vi "ConfigureIndex.vi"(0 "Axis In":T7, 1 "Additional Settings":T4={"Next Index"=0, "Termination"=0, "Count"=1} {"Termination" items=["Stop", "Start Another Immediately", "Start Another x/start Index Input", "Start Another Index Without Stopping"]}, 5 "Index (0)":T6, 7 "Position":dbl, 11 "error in (no error)":errorcluster, 12 "Index Settings":T1={"Type"=1, "Dwell"=0, "Velocity"=0.0, "Accel/Decel"=0.0} {"Type" items=["Incremental", "Absolute", "Registration", "Jog"]}) -> (4 "Axis Out":T7, 6 "Index (duplicate)":T6, 15 "error out":errorcluster)   [LabVIEW 2009]
doc: "Configure an index (motion) on specified axis. Any parameters left unset will be set to their default values."
uses:
  typedefs/AxisSelect_Enum.ctl
  typedefs/Ultra3000/Index_Numeric.ctl
  typedefs/Ultra3000/AdditionalIndexSettings_Cluster.ctl
  typedefs/Ultra3000/IndexTermination.ctl
  typedefs/Ultra3000/IndexSettings_Cluster.ctl
  typedefs/Ultra3000/IndexType.ctl
  typedefs/DwellTime.ctl
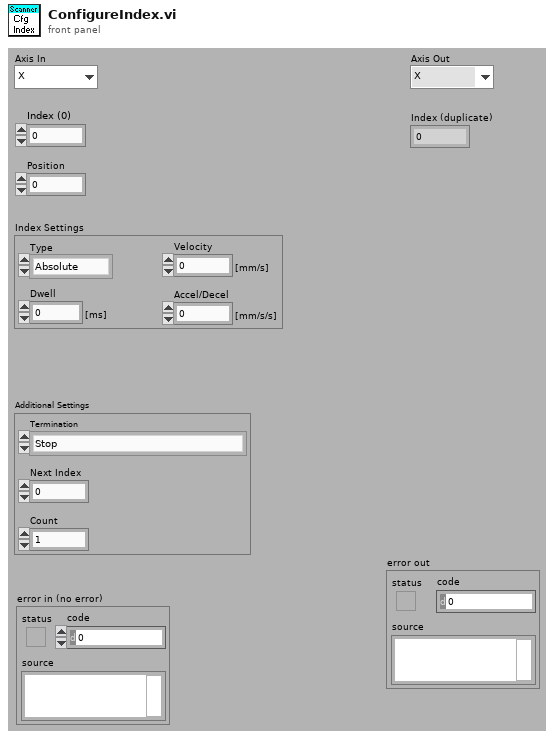
[diagram p1: front panel]
types:
  T1 = typedef "IndexSettings_Cluster.ctl" = cluster{"Type":T2, "Dwell":T3, "Velocity":dbl, "Accel/Decel":dbl}
  T2 = typedef "IndexType.ctl" = i32
  T3 = typedef "DwellTime.ctl" = u16
  T4 = typedef "AdditionalIndexSettings_Cluster.ctl" = cluster{"Next Index":u8, "Termination":T5, "Count":u16}
  T5 = typedef "IndexTermination.ctl" = i32
  T6 = typedef "Index_Numeric.ctl" = u8
  T7 = typedef "AxisSelect_Enum.ctl" = enum16{"X", "Y", "Z", "Axis Space"}
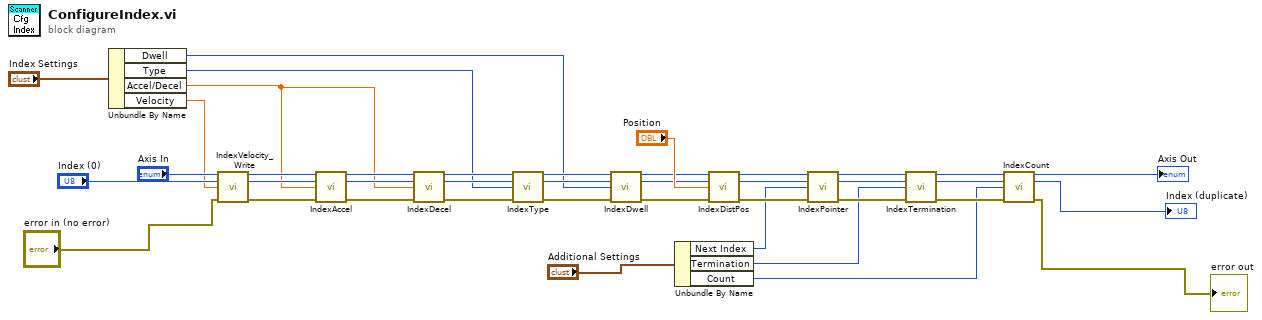
[diagram p0: block diagram]
diagram:
  n1 = Unbundle By Name("Index Settings") -> ("Dwell"=w6:T3, "Type"=w19:T2, "Accel/Decel"=w20:dbl, "Velocity"=w21:dbl)
  n2 = call "IndexVelocity_Write.vi"("Axis In"="Axis In", "Index (0)"="Index (0)", "Velocity"=w21, "error in (no error)"="error in (no error)") -> ("Axis Out"=w29:T7, "Index (duplicate)"=w26:T6, "error out"=w36:errorcluster)  [unwired: 9 in]
  n3 = call "IndexAccel.vi"("Axis In"=w29, "Index (0)"=w26, "Acceleration"=w20, "error in (no error)"=w36) -> ("Axis Out"=w30:T7, "Index (duplicate)"=w25:T6, "error out"=w37:errorcluster)  [unwired: 9 in]
  n4 = call "IndexDecel.vi"("Axis In"=w30, "Index (0)"=w25, "Deceleration"=w20, "error in (no error)"=w37) -> ("Axis Out"=w31:T7, "Index (duplicate)"=w24:T6, "error out"=w38:errorcluster)  [unwired: 9 in]
  n5 = call "IndexType.vi"("Axis In"=w31, "Index (0)"=w24, "Index Type"=w19, "error in (no error)"=w38) -> ("Axis Out"=w18:T7, "Index (duplicate)"=w17:T6, "error out"=w16:errorcluster)  [unwired: 9 in]
  n6 = call "IndexDwell.vi"("Axis In"=w18, "Index (0)"=w17, "Dwell (ms)"=w6, "error in (no error)"=w16) -> ("Axis Out"=w13:T7, "Index (duplicate)"=w14:T6, "error out"=w15:errorcluster)  [unwired: 9 in]
  n7 = Unbundle By Name("Additional Settings") -> ("Next Index"=w9:u8, "Termination"=w8:T5, "Count"=w7:u16)
  n8 = call "IndexDistPos.vi"("Axis In"=w13, "Index (0)"=w14, "Position"="Position", "error in (no error)"=w15) -> ("Axis Out"=w35:T7, "Index (duplicate)"=w32:T6, "error out"=w40:errorcluster)  [unwired: 9 in]
  n9 = call "IndexPointer.vi"("Axis In"=w35, "Index (0)"=w32, "Index Pointer"=w9, "error in (no error)"=w40) -> ("Axis Out"=w34:T7, "Index (duplicate)"=w33:T6, "error out"=w39:errorcluster)  [unwired: 9 in]
  n10 = call "IndexTermination.vi"("Axis In"=w34, "Index (0)"=w33, "Index Termination"=w8, "error in (no error)"=w39) -> ("Axis Out"=w12:T7, "Index (duplicate)"=w11:T6, "error out"=w10:errorcluster)  [unwired: 9 in]
  n11 = call "IndexCount.vi"("Axis In"=w12, "Index (0)"=w11, "Index Count"=w7, "error in (no error)"=w10) -> ("Axis Out"=→"Axis Out":T7, "Index (duplicate)"=→"Index (duplicate)":T6, "error out"=→"error out":errorcluster)  [unwired: 9 in]
